vi "Run Function.vi"(8 "error in (no error)":errorcluster, 11 "Operator UI in":refnum<class "Controller UI.lvclass">) -> (0 "error out":errorcluster, 3 "Operator UI out":refnum<class "Controller UI.lvclass">)   [LabVIEW 2016, in "Controller UI.lvlib" / "Controller UI.lvclass"]
uses:
  <userlib>/Common Components/Controller UI/Controller UI.lvclass
  C:/Program Files (x86)/National Instruments/LabVIEW 2016/vi.lib/ActorFramework/Actor/Actor.lvclass
  <vilib>/ActorFramework/Actor/Actor.lvclass/Actor.ctl
  <vilib>/ActorFramework/Message Enqueuer/Message Enqueuer.lvclass/Message Enqueuer.ctl
  <vilib>/ActorFramework/Message Enqueuer/Init from Existing Queue.vi
  <vilib>/ActorFramework/Message Enqueuer/Message Enqueuer.lvclass
  <userlib>/Common Components/Controller/Messages/Launch Functions Message/Launch Functions Message.lvclass
  <userlib>/Common Components/User Interface/Messages/Update Status Display/Update Status Display.lvclass
  <vilib>/ActorFramework/Actor/Actor.lvclass
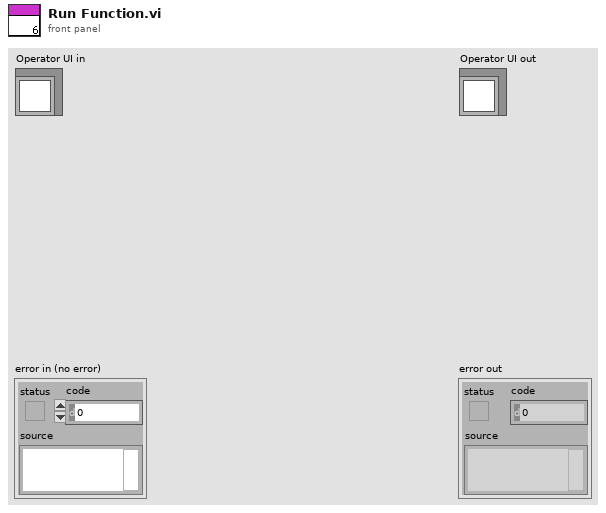
[diagram p1: front panel]
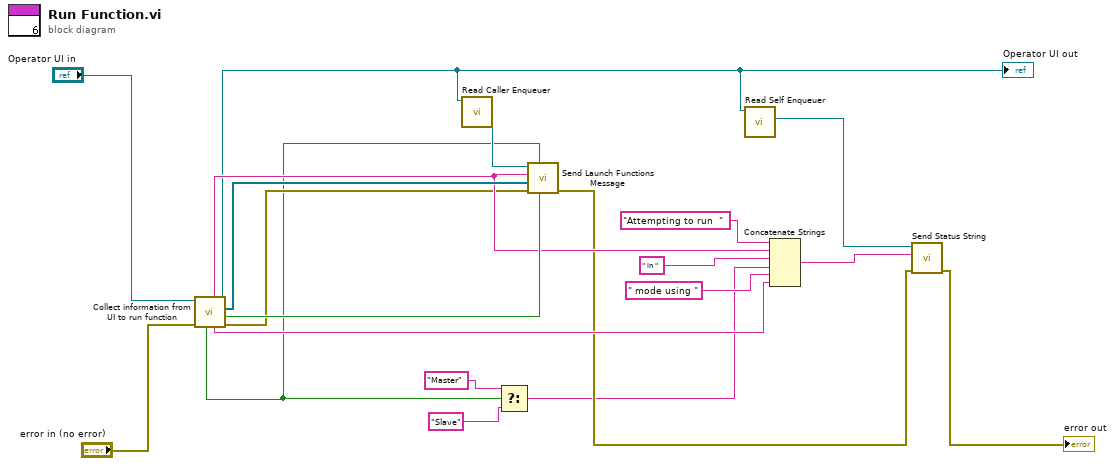
[diagram p0: block diagram]
diagram:
  n1 = call <userlib>:"Collect information from UI to run function.vi"("error in (no error)"="error in (no error)", "Function UI in"="Operator UI in") -> ("error out"=w7:errorcluster, "Show UI?"=w19:bool, "Devices"=w20:refnum<class "DevInfo.lvclass">[], "Function UI out"=w9:refnum<class "Controller UI.lvclass">, "String"=w14:string, "Function Name"=w17:string, "Master?"=w1:bool)  [unwired: 3 in]
  "Operator UI out" <- w9
  n2 = call <vilib>:"Read Caller Enqueuer.vi"("Actor"=w9) -> ("Caller Enqueuer"=w13:refnum<class "Message Enqueuer.lvclass">)  [unwired: 10 in]
  n3 = Select(t="Master", s=w1, f="Slave") -> (s? t:f=w2:string)
  n4 = call <userlib>:"Send Launch Functions Message.vi"("Show FP?"=w19, "Master?"=w1, "error in (no error)"=w7, "Device Names"=w20, "Function Name"=w17, "Self Enqueuer In"=w13) -> ("error out"=w6:errorcluster)  [unwired: 4 in, 1 out]
  n5 = call <vilib>:"Read Self Enqueuer.vi"("Actor"=w9) -> ("Self Enqueuer"=w12:refnum<class "Message Enqueuer.lvclass">)  [unwired: 10 in]
  n6 = Concatenate Strings("Attempting to run  " ("string"), w17, " in " ("string"), w2, " mode using " ("string"), w14) -> (w15:string)
  n7 = call <userlib>:"Send Status String.vi"("error in (no error)"=w6, "String"=w15, "Message Enqueuer in"=w12) -> ("error out"=→"error out":errorcluster)  [unwired: 7 in, 1 out]
